vi "DVS_LabVIEWController_one_panel - Copy.vi"() -> ()   [LabVIEW 2013]
doc: "This example demonstrates temperature control and monitoring.\n\nNote:\nBefore start this VI is it necessary:\n\n- preconfigure some specific parameters that are not supported by this driver (e.g. PV-I/O Type, Linearization type, Alarm Input Values... ) by Quick Codes, or by Eurotherm iTools or by instrument front panel controls\n- enter correct VISA Resource Descriptor, Device Address and Baud Rate into front-panel controls"
uses:
  <vilib>/Utility/file.llb/Write To Spreadsheet File (string).vi
  <vilib>/Instr/_visa.llb/VISA Configure Serial Port (Instr).vi
  <instrlib>/Keithley 24XX/Public/Data/Read (Single Point).vi
  <instrlib>/Keithley 24XX/Keithley 24XX.lvlib
panel:
  in  "Automatically stop measurement?":bool
  in  "Stop after":dbl
  out "min remaining":dbl
  in  "stop":bool
  in  "Add comments to the   here and click anywhere outside\nthe comment box to save. The time at which the comment is\nsaved is recorded in the data file.":string
  out "Program Errors":errorcluster
  in  "O2 PUMP":bool
  in  "QCM":bool
  in  "Keithley 2420":bool
  in  "J-KEM":bool
  in  "RapidOX":bool
  out "Starting Time":string
  out "Time Elapsed (min)":dbl caption="Elapsed Time (s)"
  out "Frequency (Hz)":dbl format="%.6e"
  out "Resistance (Ohm)":dbl format="%.6e"
  out "Waveform Chart 7":T1(graph)
  out "Current Temp (C)":dbl
  in  "Setpoint (C)":dbl=25.0
  out "Current Setpoint (C)":dbl
  out "Waveform Chart 5":cluster{dbl, dbl}(graph)
  out "Waveform Chart":cluster{dbl}(graph)
  out "Torr":dbl
  out "%":dbl
  out "atm":dbl
  in  "Com Port":i32(ring) items=["Com 1", "Com 2", "Com 3", "Com 4", "Com 5", "Com 6", "COM 7", "COM 8", "COM 9", "COM 10", "COM 11", "COM 12", "com 13", "COM 14"]
  in  "Baud Rate 2":i32(ring)=2 items=["2400", "4800", "9600", "19200", "38400", "57600", "115200"]
  in  "Com Port 2":i32(ring) items=["Com 1", "Com 2", "Com 3", "Com 4", "Com 5", "Com 6", "COM 7", "COM 8", "COM 9", "COM 10", "COM 11", "COM 12", "com 13", "COM 14"]
  out "Waveform Chart 6":cluster{dbl}(graph)
  out "O2 Concentration (PPM)":dbl
  out "Resistance (Ohm)":sgl
  out "Waveform Chart 4":cluster{"Resistance":sgl}(graph)
  # "Configuring Instrument\n \nPlease Wait......\n\nChart will update in 20 sec"
  # "Instruments\nConnected:"
  # "COMMENT BOX"
  # "Errors"
  # "Setup"
  # "min"
  # "SRS QCM\nController"
  # "J-Kem Temp Control"
  # "SetNag O2 Pump"
  # "O2 Partial Pressure"
  # "Rapidox O2\nSensor"
  # "Keithley 2420\nRead Resistance"
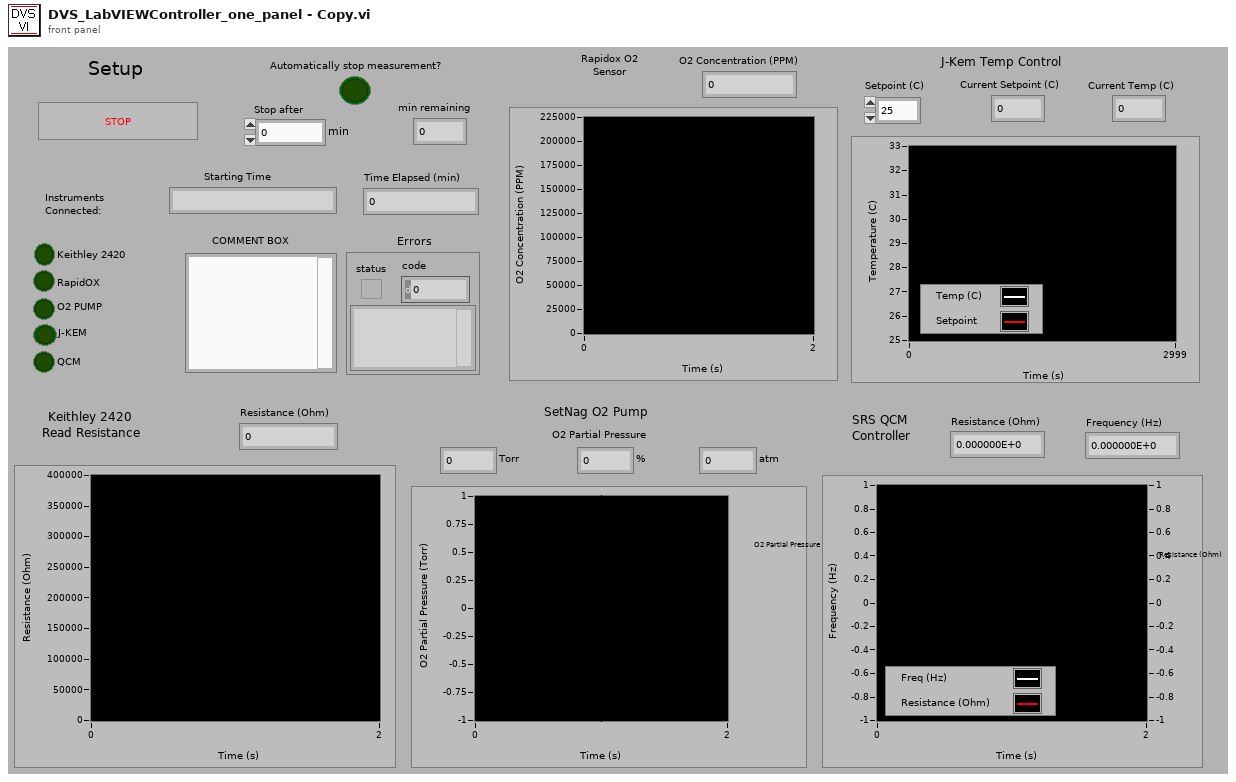
[diagram p1: front panel]
types:
  T1 = cluster{"Frequency out":dbl, "Resistance out":dbl}
  T2 = enum16{"open", "open or create", "create or replace", "create", "open (read only)"}
  T3 = enum16{"no parity", "odd parity", "even parity", "mark parity", "space parity"}
  T4 = cluster{bool, "VISA resource name":refnum<visa-resource-name>, "error out":errorcluster}
  T5 = cluster{bool, "VISA resource name out":refnum<visa-resource-name>, "error out":errorcluster}
  T6 = cluster{"Frequency out":dbl, "Resistance out":dbl}[]
  T7 = cluster{bool, "VISA out":refnum<visa-resource-name>, "error out":errorcluster}
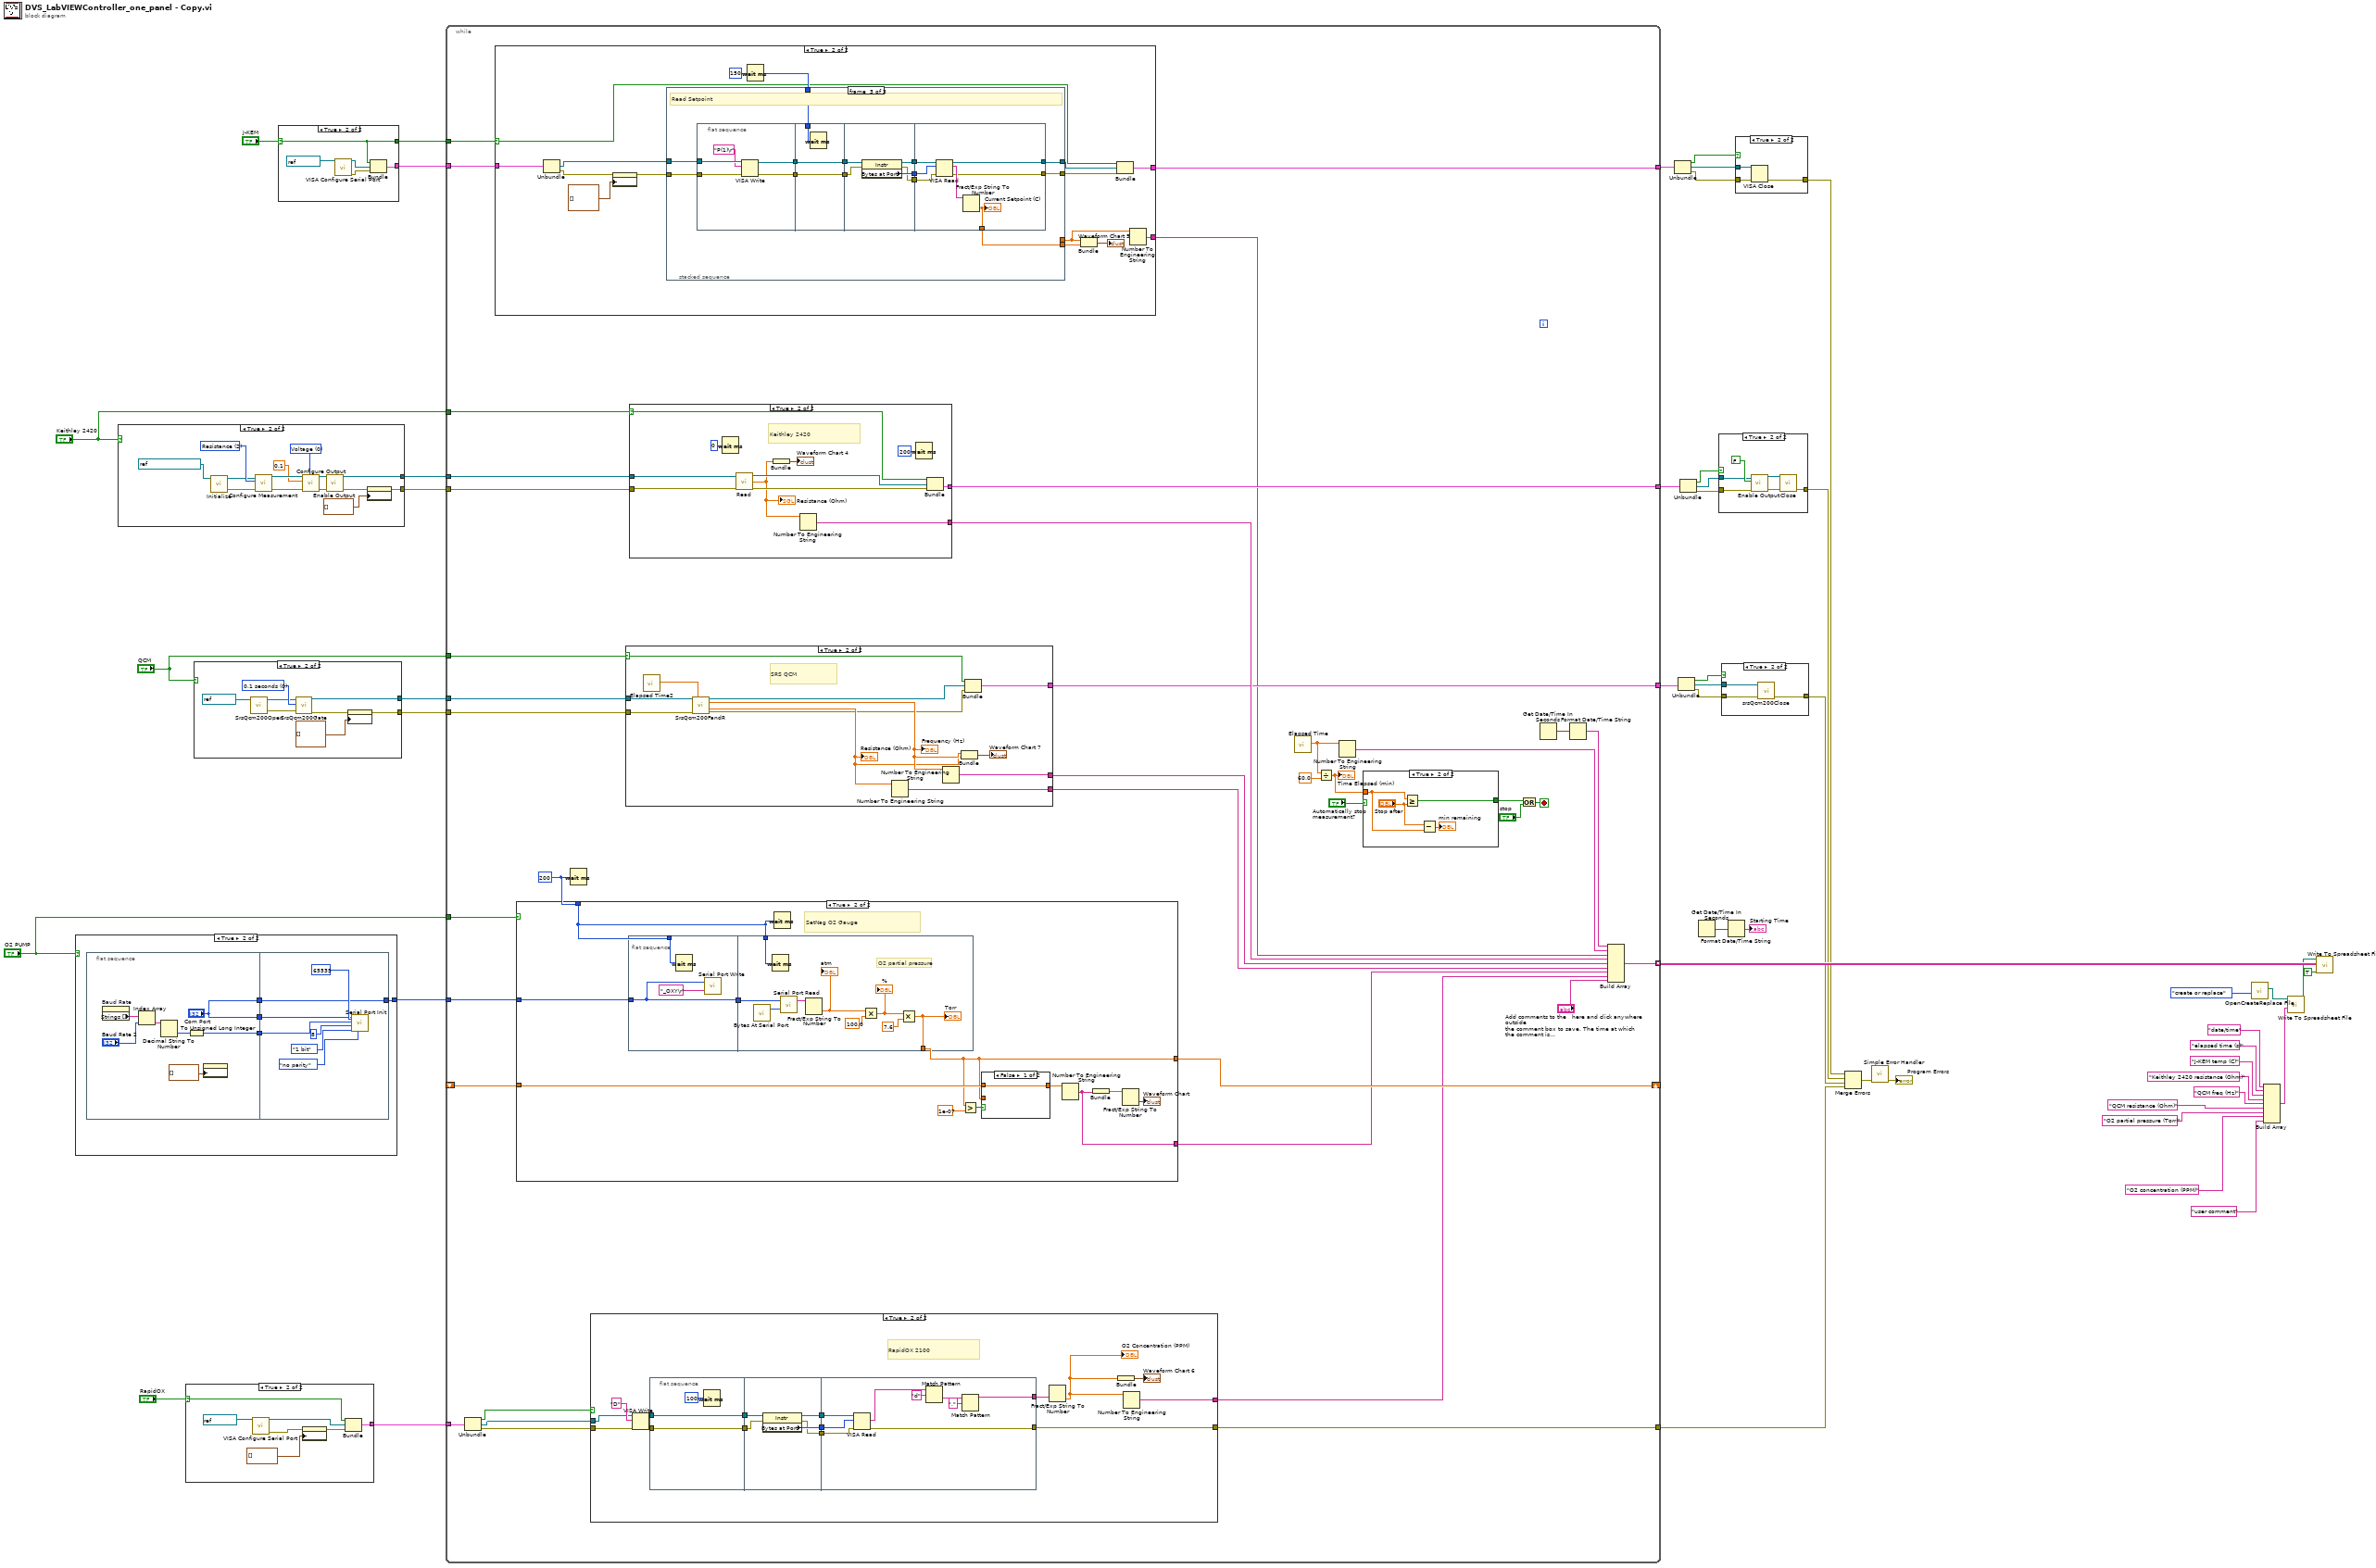
[diagram p0: block diagram]
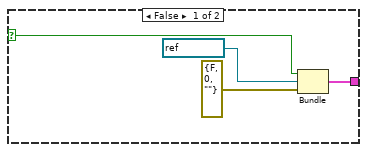
[diagram p2: hidden frame]
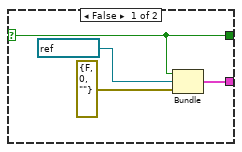
[diagram p4: hidden frame]
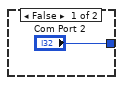
[diagram p5: hidden frame]
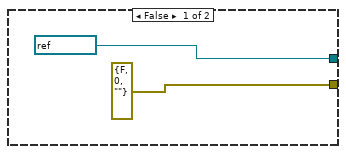
[diagram p7: hidden frame]
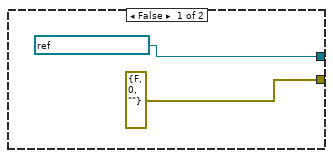
[diagram p9: hidden frame]
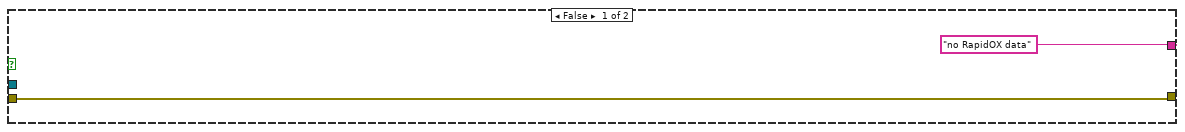
[diagram p10: hidden frame]
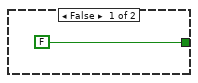
[diagram p11: hidden frame]
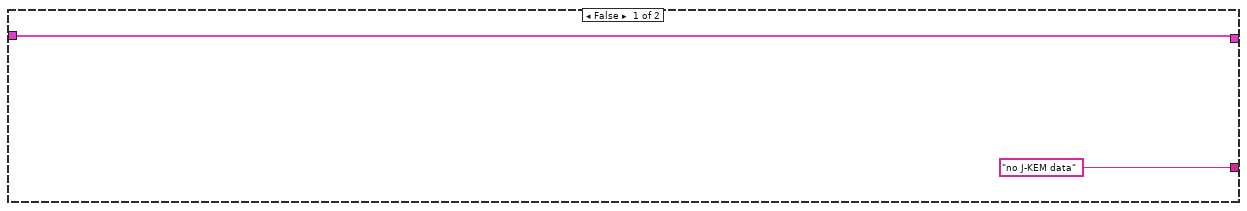
[diagram p12: hidden frame]
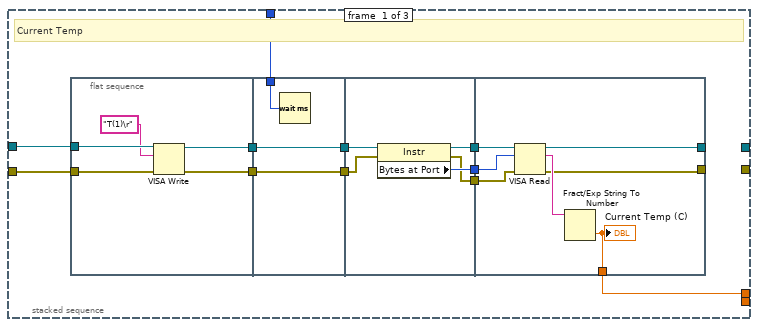
[diagram p13: hidden frame]
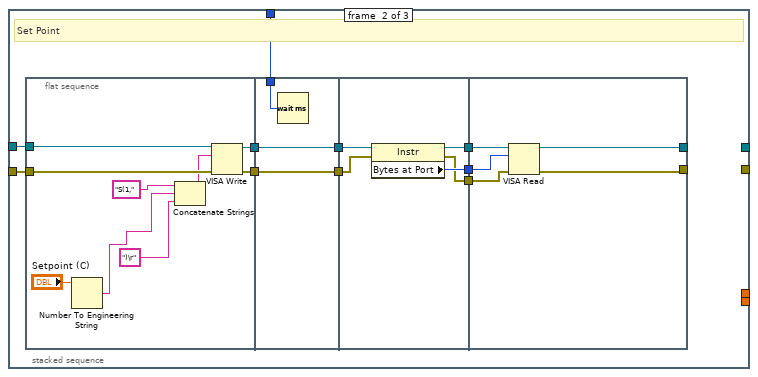
[diagram p14: hidden frame]
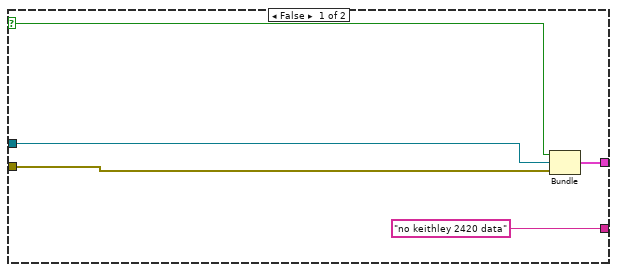
[diagram p15: hidden frame]
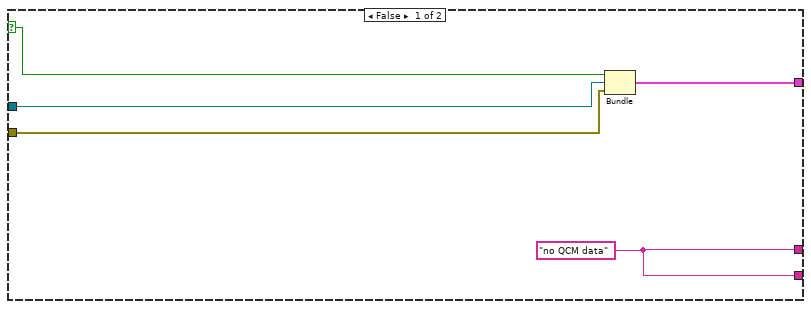
[diagram p16: hidden frame]
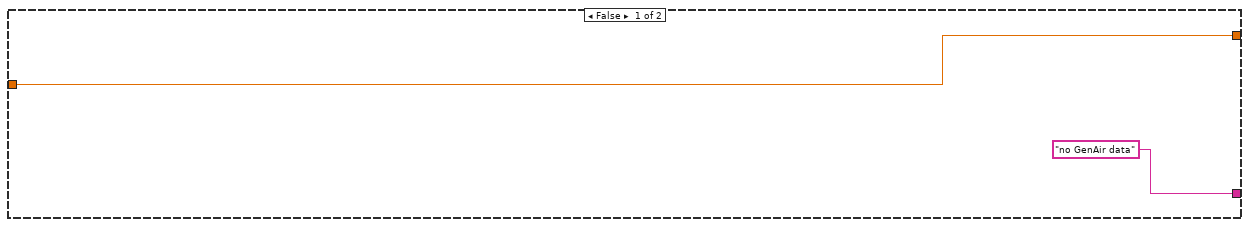
[diagram p17: hidden frame]
diagram:
  n1 = case shown="True" "O2 PUMP" {
    tunnel: ["Com Port 2" w50] -> w36
    frame False {
    }
    frame True {
      n2 = flat-sequence {
        tunnel: ["Com Port"] -> w53
        tunnel: [w56] -> w52
        tunnel: ["Com Port"] -> w51
        tunnel: w53 -> [w62]
        tunnel: w52 -> [w61]
        tunnel: w51 -> [w63]
        tunnel: [w63] -> w50
        frame #0 {
          n3 = property on="Baud Rate" class="Ring (strict)"() -> ("Strings []"=w58:string[])  [unwired: 2 in, 2 out]
          n4 = Index Array(array=w58, index="Baud Rate 2") -> (element=w59:string)
          n5 = Decimal String To Number(string=w59) -> (number=w57:i32)  [unwired: 2 in, 1 out]
          n6 = To Unsigned Long Integer(number=w57) -> (unsigned 32bit integer=w56:u32)
          n7 = property on="Waveform Chart" class="WFChart (strict)"("History Data"=cluster{dbl}[] []) -> ()  [unwired: 2 in, 2 out]
        }
        frame #1 {
          n8 = call <vilib>:"Serial Port Init.vi"("parity"=T3."no parity", "buffer size"=u16 65535, "stop bits"=enum16{"1 bit", "1.5 bits", "2 bits"}."1 bit", "data bits"=u16 8, "baud rate"=w61, "port number"=w62) -> ()  [unwired: 1 in, 1 out]
        }
      }
    }
  }
  n9 = case shown="True" "Keithley 2420" {
    tunnel: [refnum<visa-resource-name> "GPIB1::24::INSTR" ("VISA resource name") w74] -> w42
    tunnel: [errorcluster {"status"=FALSE, "code"=0, "source"=""} ("error out") w71] -> w41
    frame False {
    }
    frame True {
      w77 = u16 0 items=["Voltage", "Current"] ("Source Mode  (0: Voltage)")
      w82 = u16 2 items=["Volts", "Current", "Resistance"] ("Function (0: Volts)")
      n10 = call <instrlib>:"Initialize.vi"("VISA resource name"=refnum<visa-resource-name> "GPIB1::24::INSTR") -> ("error out"=w75:errorcluster, "VISA resource name out"=w76:refnum<visa-resource-name>)  [unwired: 9 in]
      n11 = call <instrlib>:"Configure Measurement.vi"("error in (no error)"=w75, "Function (0: Volts)"=w82, "VISA resource name"=w76) -> ("error out"=w81:errorcluster, "VISA resource name out"=w80:refnum<visa-resource-name>)  [unwired: 7 in]
      n12 = call <instrlib>:"Configure Output.vi"("Source Mode  (0: Voltage)"=w77, "error in (no error)"=w81, "Output Level (0)"=0.1 ("Output Level (V)"), "VISA resource name"=w80) -> ("error out"=w79:errorcluster, "VISA resource name out"=w78:refnum<visa-resource-name>)  [unwired: 6 in]
      n13 = call <instrlib>:"Enable Output.vi"("error in (no error)"=w79, "VISA resource name"=w78) -> ("error out"=w70:errorcluster, "VISA resource name out"=w74:refnum<visa-resource-name>)  [unwired: 8 in]
      n14 = property on="Waveform Chart 4" class="WFChart (strict)"(error in=w70, "History Data"=cluster{"Resistance":sgl}[] []) -> (error out=w71:errorcluster)  [unwired: 1 in, 1 out]
    }
  }
  n15 = case shown="True" "RapidOX" {
    selector: "RapidOX" -> [w84 w91]
    tunnel: [w85 w92] -> w3
    frame False {
      n16 = Bundle(w84, "VISA resource name"=refnum<visa-resource-name> "COM7", "error out"=errorcluster {"status"=FALSE, "code"=0, "source"=""}) -> (w85:T4)  [unwired: 1 in]
    }
    frame True {
      n17 = call-poly "VISA Configure Serial Port"("VISA resource name"=refnum<visa-resource-name> "COM7") -> ("VISA resource name out"=w93:refnum<visa-resource-name>, "error out"=w89:errorcluster)  [unwired: 13 in]
      n18 = property on="Waveform Chart 6" class="WFChart (strict)"(error in=w89, "History Data"=cluster{dbl}[] []) -> (error out=w88:errorcluster)  [unwired: 1 in, 1 out]
      n19 = Bundle(w91, "VISA resource name out"=w93, "error out"=w88) -> (w92:T5)  [unwired: 1 in]
    }
  }
  n20 = case shown="True" "QCM" {
    tunnel: [refnum<visa-resource-name> "COM6" ("VISA in") w100] -> w40
    tunnel: [errorcluster {"status"=FALSE, "code"=0, "source"=""} ("error out") w98] -> w39
    frame False {
    }
    frame True {
      w104 = u16 0 items=["0.1 seconds", "1.0 seconds", "10.0 seconds"] ("Gate in")
      n21 = call <instrlib>:"SrsQcm200Open.vi"("VISA in"=refnum<visa-resource-name> "COM6") -> ("error out"=w101:errorcluster, "VISA out"=w102:refnum<visa-resource-name>)  [unwired: 4 in]
      n22 = call <instrlib>:"SrsQcm200Gate.vi"("VISA in"=w102, "Gate in"=w104, "error in (no error)"=w101) -> ("VISA out"=w100:refnum<visa-resource-name>, "error out"=w97:errorcluster)  [unwired: 14 in, 1 out]
      n23 = property on="Waveform Chart 7" class="WFChart (strict)"(error in=w97, "History Data"=T6 []) -> (error out=w98:errorcluster)  [unwired: 1 in, 1 out]
    }
  }
  n24 = case shown="True" "J-KEM" {
    selector: "J-KEM" -> [w105 w109]
    tunnel: [w106 w110] -> w25
    tunnel: [w105 w109] -> w18
    frame False {
      n25 = Bundle(w105, "VISA resource name"=refnum<visa-resource-name> "COM3", "error out"=errorcluster {"status"=FALSE, "code"=0, "source"=""}) -> (w106:T4)  [unwired: 1 in]
    }
    frame True {
      n26 = call-poly "VISA Configure Serial Port"("VISA resource name"=refnum<visa-resource-name> "COM3") -> ("VISA resource name out"=w112:refnum<visa-resource-name>, "error out"=w111:errorcluster)  [unwired: 13 in]
      n27 = Bundle(w109, "VISA resource name out"=w112, "error out"=w111) -> (w110:T5)  [unwired: 1 in]
    }
  }
  n28 = while {
    shift-right: [w150] -> _
    shift-left: _ -> [w149]
    tunnel: [w146] -> w44 mode=indexing
    tunnel: "Keithley 2420" -> [w142]
    tunnel: w42 -> [w144]
    tunnel: w41 -> [w143]
    tunnel: w40 -> [w141]
    tunnel: w39 -> [w140]
    tunnel: "QCM" -> [w138]
    tunnel: "O2 PUMP" -> [w131]
    tunnel: w36 -> [w137]
    tunnel: [w133] -> w33
    tunnel: [w132] -> w29
    tunnel: w25 -> [w130]
    tunnel: [w129] -> w23
    tunnel: w18 -> [w127]
    tunnel: w3 -> [w119]
    tunnel: [w114] -> w1
    stop <- w125 stop-if-true
    w148 = u32 200 ("milliseconds to wait")
    n29 = Unbundle(w119) -> (w118:bool, "VISA resource name out"=w117:refnum<visa-resource-name>, "error out"=w116:errorcluster)
    n30 = case shown="True" w127 {
      selector: w127 -> [_ w197]
      tunnel: w130 -> [w193 w202]
      tunnel: [w193 w200] -> w129
      tunnel: ["no J-KEM data" w198] -> w128
      frame False {
      }
      frame True {
        w207 = u32 150 ("milliseconds to wait")
        n31 = Unbundle(w202) -> ("VISA resource name out"=w201:refnum<visa-resource-name>, "error out"=w195:errorcluster)  [unwired: 1 out]
        n32 = property on="Waveform Chart 5" class="WFChart (strict)"(error in=w195, "History Data"=cluster{dbl, dbl}[] []) -> (error out=w194:errorcluster)  [unwired: 1 in, 1 out]
        n33 = stacked-sequence {
          tunnel: w201 -> [w211 w241 w275]
          tunnel: w194 -> [w210 w240 w274]
          tunnel: w207 -> [w209 w239 w276]
          tunnel: [_ _ w273] -> w203
          tunnel: [_ _ w272] -> w204
          tunnel: [w208 _ _] -> w199
          tunnel: [_ _ w271] -> w206
          frame #0 {
            # "Current Temp"
            n34 = flat-sequence {
              tunnel: w211 -> [w223]
              tunnel: w210 -> [w222]
              tunnel: [w220] -> w218
              tunnel: [w219] -> w217
              tunnel: w209 -> [w226]
              tunnel: [w225] -> w216
              tunnel: w218 -> [w225]
              tunnel: w217 -> [w224]
              tunnel: [w224] -> w215
              tunnel: w216 -> [w231]
              tunnel: w215 -> [w230]
              tunnel: [w229] -> w214
              tunnel: [w228] -> w213
              tunnel: [w227] -> w212
              tunnel: w214 -> [w238]
              tunnel: w213 -> [w237]
              tunnel: w212 -> [w236]
              tunnel: [w233] -> _
              tunnel: [w234] -> _
              tunnel: [w232] -> w208
              frame #0 {
                n35 = VISA Write(VISA resource name=w223, write buffer="T(1)\r", error in (no error)=w222) -> (VISA resource name out=w220:refnum<visa-resource-name>, error out=w219:errorcluster)  [unwired: 1 out]
              }
              frame #1 {
                n36 = Wait (ms)(milliseconds to wait=w226) -> ()  [unwired: 1 out]
              }
              frame #2 {
                n37 = property class="Instr"(reference=w231, error in=w230) -> (reference out=w229:refnum<visa-resource-name>, error out=w227:errorcluster, "Bytes at Port"=w228:u32)
              }
              frame #3 {
                n38 = VISA Read(VISA resource name=w238, byte count=w237, error in (no error)=w236) -> (VISA resource name out=w234:refnum<visa-resource-name>, read buffer=w235:string, error out=w233:errorcluster)  [unwired: 1 out]
                n39 = Fract/Exp String To Number(string=w235) -> (number=w232:dbl)  [unwired: 3 in, 1 out]
                "Current Temp (C)" <- w232
              }
            }
          }
          frame #1 {
            # "Set Point"
            n40 = flat-sequence {
              tunnel: w241 -> [w257]
              tunnel: w240 -> [w256]
              tunnel: [w255] -> w248
              tunnel: [w254] -> w247
              tunnel: w239 -> [w260]
              tunnel: [w259] -> w246
              tunnel: w248 -> [w259]
              tunnel: w247 -> [w258]
              tunnel: [w258] -> w245
              tunnel: w246 -> [w265]
              tunnel: w245 -> [w264]
              tunnel: [w263] -> w244
              tunnel: [w262] -> w243
              tunnel: [w261] -> w242
              tunnel: w244 -> [w270]
              tunnel: w243 -> [w269]
              tunnel: w242 -> [w268]
              tunnel: [w266] -> _
              tunnel: [w267] -> _
              frame #0 {
                n41 = Number To Engineering String(4:"Setpoint (C)") -> (0:w250:string)  [unwired: 3 in]
                n42 = Concatenate Strings("S(1," ("write buffer"), w250, ")\r" ("write buffer")) -> (w253:string)
                n43 = VISA Write(VISA resource name=w257, write buffer=w253, error in (no error)=w256) -> (VISA resource name out=w255:refnum<visa-resource-name>, error out=w254:errorcluster)  [unwired: 1 out]
              }
              frame #1 {
                n44 = Wait (ms)(milliseconds to wait=w260) -> ()  [unwired: 1 out]
              }
              frame #2 {
                n45 = property class="Instr"(reference=w265, error in=w264) -> (reference out=w263:refnum<visa-resource-name>, error out=w261:errorcluster, "Bytes at Port"=w262:u32)
              }
              frame #3 {
                n46 = VISA Read(VISA resource name=w270, byte count=w269, error in (no error)=w268) -> (VISA resource name out=w267:refnum<visa-resource-name>, error out=w266:errorcluster)  [unwired: 2 out]
              }
            }
          }
          frame #2 {
            # "Read Setpoint"
            n47 = flat-sequence {
              tunnel: w275 -> [w288]
              tunnel: w274 -> [w287]
              tunnel: [w285] -> w283
              tunnel: [w284] -> w282
              tunnel: [w291] -> w281
              tunnel: w283 -> [w291]
              tunnel: w282 -> [w290]
              tunnel: [w290] -> w280
              tunnel: w276 -> [w289]
              tunnel: w281 -> [w296]
              tunnel: w280 -> [w295]
              tunnel: [w294] -> w279
              tunnel: [w293] -> w278
              tunnel: [w292] -> w277
              tunnel: w279 -> [w303]
              tunnel: w278 -> [w302]
              tunnel: w277 -> [w301]
              tunnel: [w298] -> w272
              tunnel: [w299] -> w273
              tunnel: [w297] -> w271
              frame #0 {
                n48 = VISA Write(VISA resource name=w288, write buffer="P(1)\r", error in (no error)=w287) -> (VISA resource name out=w285:refnum<visa-resource-name>, error out=w284:errorcluster)  [unwired: 1 out]
              }
              frame #1 {
                n49 = Wait (ms)(milliseconds to wait=w289) -> ()  [unwired: 1 out]
              }
              frame #2 {
                n50 = property class="Instr"(reference=w296, error in=w295) -> (reference out=w294:refnum<visa-resource-name>, error out=w292:errorcluster, "Bytes at Port"=w293:u32)
              }
              frame #3 {
                n51 = VISA Read(VISA resource name=w303, byte count=w302, error in (no error)=w301) -> (VISA resource name out=w299:refnum<visa-resource-name>, read buffer=w300:string, error out=w298:errorcluster)  [unwired: 1 out]
                n52 = Fract/Exp String To Number(string=w300) -> (number=w297:dbl)  [unwired: 3 in, 1 out]
                "Current Setpoint (C)" <- w297
              }
            }
          }
        }
        n53 = Wait (ms)(milliseconds to wait=w207) -> ()  [unwired: 1 out]
        n54 = Bundle(w199, w206) -> (→"Waveform Chart 5":cluster{dbl, dbl})  [unwired: 1 in]
        n55 = Bundle(w197, "VISA resource name out"=w203, "error out"=w204) -> (w200:T5)  [unwired: 1 in]
        n56 = Number To Engineering String(4:w199) -> (0:w198:string)  [unwired: 3 in]
      }
    }
    n57 = case shown="True" w131 {
      tunnel: [w338 w342] -> w150
      tunnel: w149 -> [w338 w343]
      tunnel: w148 -> [_ w339]
      tunnel: w137 -> [_ w341]
      tunnel: ["no GenAir data" w340] -> w136
      frame False {
      }
      frame True {
        # "SetNag O2 Gauge"
        n58 = flat-sequence {
          tunnel: [w352] -> w349
          tunnel: w339 -> [w354]
          tunnel: w341 -> [w352]
          tunnel: w349 -> [w355]
          tunnel: w339 -> [w362]
          tunnel: [w358] -> w342
          frame #0 {
            n59 = Wait (ms)(milliseconds to wait=w354) -> ()  [unwired: 1 out]
            n60 = call <vilib>:"Serial Port Write.vi"("string to write"="_OXY\r" ("O2 partial press"), "port number"=w352) -> ()  [unwired: 1 out]
          }
          frame #1 {
            # "O2 partial pressure"
            n61 = call <vilib>:"Bytes At Serial Port.vi"() -> ("byte count"=w363:u32)  [unwired: 1 in, 1 out]
            n62 = Wait (ms)(milliseconds to wait=w362) -> ()  [unwired: 1 out]
            n63 = call <vilib>:"Serial Port Read.vi"("requested byte count"=w363, "port number"=w355) -> ("string read"=w361:string)  [unwired: 1 out]
            n64 = Fract/Exp String To Number(string=w361) -> (number=w359:dbl)  [unwired: 3 in, 1 out]
            "atm" <- w359
            n65 = Multiply(x=w359, y=100.0) -> (x*y=w356:dbl)
            "%" <- w356
            n66 = Multiply(x=w356, y=7.6) -> (x*y=w358:dbl)
            "Torr" <- w358
          }
        }
        n67 = Wait (ms)(milliseconds to wait=w339) -> ()  [unwired: 1 out]
        n68 = Greater?(x=w342, y=1e-07) -> (0:w345:bool)
        n69 = case shown="False" w345 {
          tunnel: [w350 w351] -> w344
          tunnel: w342 -> [_ w351]
          tunnel: w343 -> [w350 _]
          frame False {
          }
          frame True {
          }
        }
        n70 = Number To Engineering String(4:w344) -> (0:w340:string)  [unwired: 3 in]
        n71 = Bundle(w340) -> (w347:cluster{string})  [unwired: 1 in]
        n72 = Fract/Exp String To Number(string=w347) -> (number=→"Waveform Chart":cluster{dbl})  [unwired: 3 in, 1 out]
      }
    }
    n73 = Wait (ms)(milliseconds to wait=w148) -> ()  [unwired: 1 out]
    n74 = case shown="True" w118 {
      tunnel: w117 -> [_ w160]
      tunnel: w116 -> [w153 w159]
      tunnel: ["no RapidOX data" w158] -> w115
      tunnel: [w153 w155] -> w114
      frame False {
      }
      frame True {
        # "RapidOX 2100"
        n75 = VISA Write(VISA resource name=w160, write buffer="D", error in (no error)=w159) -> (VISA resource name out=w163:refnum<visa-resource-name>, error out=w162:errorcluster)  [unwired: 1 out]
        n76 = flat-sequence {
          tunnel: [w172] -> w169
          tunnel: [w170] -> w168
          tunnel: w163 -> [w172]
          tunnel: w162 -> [w170]
          tunnel: w169 -> [w177]
          tunnel: w168 -> [w176]
          tunnel: [w175] -> w167
          tunnel: [w174] -> w166
          tunnel: [w173] -> w165
          tunnel: w167 -> [w186]
          tunnel: w166 -> [w185]
          tunnel: w165 -> [w184]
          tunnel: [w183] -> w155
          tunnel: [w178] -> w157
          frame #0 {
            n77 = Wait (ms)(milliseconds to wait=u32 100) -> ()  [unwired: 1 out]
          }
          frame #1 {
            n78 = property class="Instr"(reference=w177, error in=w176) -> (reference out=w175:refnum<visa-resource-name>, error out=w173:errorcluster, "Bytes at Port"=w174:u32)
          }
          frame #2 {
            n79 = VISA Read(VISA resource name=w186, byte count=w185, error in (no error)=w184) -> (read buffer=w181:string, error out=w183:errorcluster)  [unwired: 2 out]
            n80 = Match Pattern(string=w181, regular expression="d") -> (after substring=w179:string)  [unwired: 1 in, 3 out]
            n81 = Match Pattern(string=w179, regular expression=",") -> (before substring=w178:string)  [unwired: 1 in, 3 out]
          }
        }
        n82 = Fract/Exp String To Number(string=w157) -> (number=w156:dbl)  [unwired: 3 in, 1 out]
        "O2 Concentration (PPM)" <- w156
        n83 = Bundle(w156) -> (→"Waveform Chart 6":cluster{dbl})  [unwired: 1 in]
        n84 = Number To Engineering String(4:w156) -> (0:w158:string)  [unwired: 3 in]
      }
    }
    n85 = case shown="True" w138 {
      selector: w138 -> [w323 w330]
      tunnel: w141 -> [w322 w335]
      tunnel: w140 -> [w321 w334]
      tunnel: [w324 w333] -> w139
      tunnel: [w324 w332] -> w135
      tunnel: [w320 w329] -> w132
      frame False {
        w324 = "no QCM data"
        n86 = Bundle(w323, "VISA out"=w322, "error out"=w321) -> (w320:T7)  [unwired: 1 in]
      }
      frame True {
        # "SRS QCM"
        n87 = call "Elapsed Time2"() -> ("Elapsed Time (s)"=w336:dbl)  [unwired: 12 in, 7 out]
        n88 = call <instrlib>:"SrsQcm200FandR.vi"("VISA in"=w335, "Reference time in"=w336, "error in (no error)"=w334) -> ("VISA out"=w331:refnum<visa-resource-name>, "Frequency out"=w327:dbl, "Resistance out"=w326:dbl, "error out"=w325:errorcluster)  [unwired: 6 in, 3 out]
        "Frequency (Hz)" <- w327
        "Resistance (Ohm)" <- w326
        n89 = Number To Engineering String(4:w326) -> (0:w332:string)  [unwired: 3 in]
        n90 = Number To Engineering String(4:w327) -> (0:w333:string)  [unwired: 3 in]
        n91 = Bundle("Frequency out"=w327, "Resistance out"=w326) -> (→"Waveform Chart 7":T1)  [unwired: 1 in]
        n92 = Bundle(w330, "VISA out"=w331, "error out"=w325) -> (w329:T7)  [unwired: 1 in]
      }
    }
    n93 = case shown="True" w142 {
      selector: w142 -> [w307 w315]
      tunnel: w144 -> [w306 w317]
      tunnel: w143 -> [w305 w309]
      tunnel: [w304 w313] -> w133
      tunnel: ["no keithley 2420 data" w312] -> w134
      frame False {
        n94 = Bundle(w307, "VISA resource name out"=w306, "error out"=w305) -> (w304:T5)  [unwired: 1 in]
      }
      frame True {
        # "Keithley 2420"
        n95 = Wait (ms)(milliseconds to wait=u32 0) -> ()  [unwired: 1 out]
        n96 = call-poly <instrlib>:"Read.vi"("VISA resource name"=w317, "error in (no error)"=w309) -> ("VISA resource name out"=w316:refnum<visa-resource-name>, "Resistance"=w310:sgl, "error out"=w314:errorcluster)  [unwired: 7 in, 4 out]
        "Resistance (Ohm)" <- w310
        n97 = Bundle("Resistance"=w310) -> (→"Waveform Chart 4":cluster{"Resistance":sgl})  [unwired: 1 in]
        n98 = Number To Engineering String(4:w310) -> (0:w312:string)  [unwired: 3 in]
        n99 = Wait (ms)(milliseconds to wait=u32 200) -> ()  [unwired: 1 out]
        n100 = Bundle(w315, "VISA resource name out"=w316, "error out"=w314) -> (w313:T5)  [unwired: 1 in]
      }
    }
    n101 = call "Elapsed Time"() -> ("Elapsed Time (s)"=w124:dbl)  [unwired: 12 in, 7 out]
    n102 = Divide(x=w124, y=60.0) -> (x/y=w122:dbl)
    "Time Elapsed (min)" <- w122
    n103 = Number To Engineering String(4:w124) -> (0:w151:string)  [unwired: 3 in]
    n104 = case shown="True" "Automatically stop measurement?" {
      tunnel: w122 -> [_ w189]
      tunnel: [FALSE w191] -> w120
      frame False {
      }
      frame True {
        n105 = Greater Or Equal?(x=w189, y="Stop after") -> (x >= y?=w191:bool)
        n106 = Subtract(x="Stop after", y=w189) -> (x-y=→"min remaining":dbl)
      }
    }
    n107 = Or(x=w120, y="stop") -> (x .or. y?=w125:bool)
    n108 = Get Date/Time In Seconds() -> (seconds since 1Jan1904=w152:timestamp)
    n109 = Format Date/Time String(seconds (now)=w152) -> (date/time string=w145:string)  [unwired: 2 in]
    n110 = Build Array(w145, w151, w128, w134, w139, w135, w136, w115, "Add comments to the   here and click anywhere outside\nthe comment box to save. The time at which the comment is\nsaved is recorded in the data file.") -> (w146:string[])
  }
  n111 = Unbundle(w23) -> (w22:bool, "VISA resource name out"=w21:refnum<visa-resource-name>, "error out"=w20:errorcluster)
  n112 = Unbundle(w29) -> (w28:bool, "VISA out"=w27:refnum<visa-resource-name>, "error out"=w26:errorcluster)
  n113 = Unbundle(w33) -> (w32:bool, "VISA resource name out"=w31:refnum<visa-resource-name>, "error out"=w30:errorcluster)
  n114 = Get Date/Time In Seconds() -> (seconds since 1Jan1904=w47:timestamp)
  n115 = case shown="True" w32 {
    tunnel: w31 -> [_ w367]
    tunnel: w30 -> [w364 w366]
    tunnel: [w364 w365] -> w34
    frame False {
    }
    frame True {
      n116 = call <instrlib>:"Enable Output.vi"("error in (no error)"=w366, "Enable Output (T: Enable)"=FALSE, "VISA resource name"=w367) -> ("error out"=w368:errorcluster, "VISA resource name out"=w370:refnum<visa-resource-name>)  [unwired: 7 in]
      n117 = call <instrlib>:"Close.vi"("error in (no error)"=w368, "VISA resource name"=w370) -> ("error out"=w365:errorcluster)  [unwired: 9 in]
    }
  }
  n118 = case shown="True" w28 {
    tunnel: w26 -> [w371 w374]
    tunnel: [w371 w373] -> w35
    tunnel: w27 -> [_ w372]
    frame False {
    }
    frame True {
      n119 = call <instrlib>:"srsQcm200Close.vi"("error in"=w374, "Visa in"=w372) -> ("error out"=w373:errorcluster)  [unwired: 3 in]
    }
  }
  n120 = Format Date/Time String(seconds (now)=w47) -> (date/time string=→"Starting Time":string)  [unwired: 2 in]
  n121 = case shown="True" w22 {
    tunnel: w21 -> [_ w378]
    tunnel: w20 -> [w375 w377]
    tunnel: [w375 w376] -> w19
    frame False {
    }
    frame True {
      n122 = VISA Close(VISA resource name=w378, error in (no error)=w377) -> (error out=w376:errorcluster)
    }
  }
  n123 = Merge Errors(w19, w34, w35, w1) -> (w45:errorcluster)
  n124 = call <vilib>:"Simple Error Handler.vi"("error in (no error)"=w45) -> ("error out"=→"Program Errors":errorcluster)  [unwired: 4 in, 4 out]
  n125 = call <instrlib>:"OpenCreateReplace File.vi"("function (open:0)"=T2."create or replace") -> ("new file path"=w7:path)  [unwired: 7 in, 3 out]
  n126 = Build Array("date/time", "elapsed time (s)", "J-KEM temp (C)", "Keithley 2420 resistance (Ohm)" ("element"), "QCM freq (Hz)", "QCM resistance (Ohm)", "O2 partial pressure (Torr)" ("element"), "O2 concentration (PPM)" ("element"), "user comment" ("element")) -> (w10:string[])
  n127 = call-poly <vilib>:"Write To Spreadsheet File.vi"("1D data"=w10, "file path (dialog if empty)"=w7) -> ("new file path (Not A Path if cancelled)"=w11:path)  [unwired: 6 in]
  n128 = call-poly <vilib>:"Write To Spreadsheet File.vi"("append to file? (new file:F)"=TRUE, "2D data"=w44, "file path (dialog if empty)"=w11) -> ()  [unwired: 5 in, 1 out]
